vi "Gradient Plot_Raw Image.vi"(8 "error in":errorcluster, 11 "Pixel Column Number":i32=390) -> (0 "error out":errorcluster, 1 "Pixel vs Gradient Graph":cluster{"Y":dbl[], "Y":dbl[]}[](graph), 2 "Pixel vs Intensity Graph":cluster{"Y":dbl[], "Y":dbl[]}[](graph), 3 "Pixel Value":i32, 5 "Maximum Gradient":u8)   [LabVIEW 2016]
uses:
  <vilib>/userdefined/High Color/IMAQdx.ctl
  <vilib>/vision/driver/NI_Vision_Acquisition_Software.lvlib
  <vilib>/vision/NI_Vision_Development_Module.lvlib
panel:
  out "Gradient Array":u8[](array[numeric])
  out "i Array":u8[](array[numeric])
  out "i+1 Array":u8[](array[numeric])
  out "Actual array":u8[](array[numeric])
  out "size(s)":i32
  out "Pixels (U8)":u8[](array[numeric])
  out "Image":T1(plugin-control)
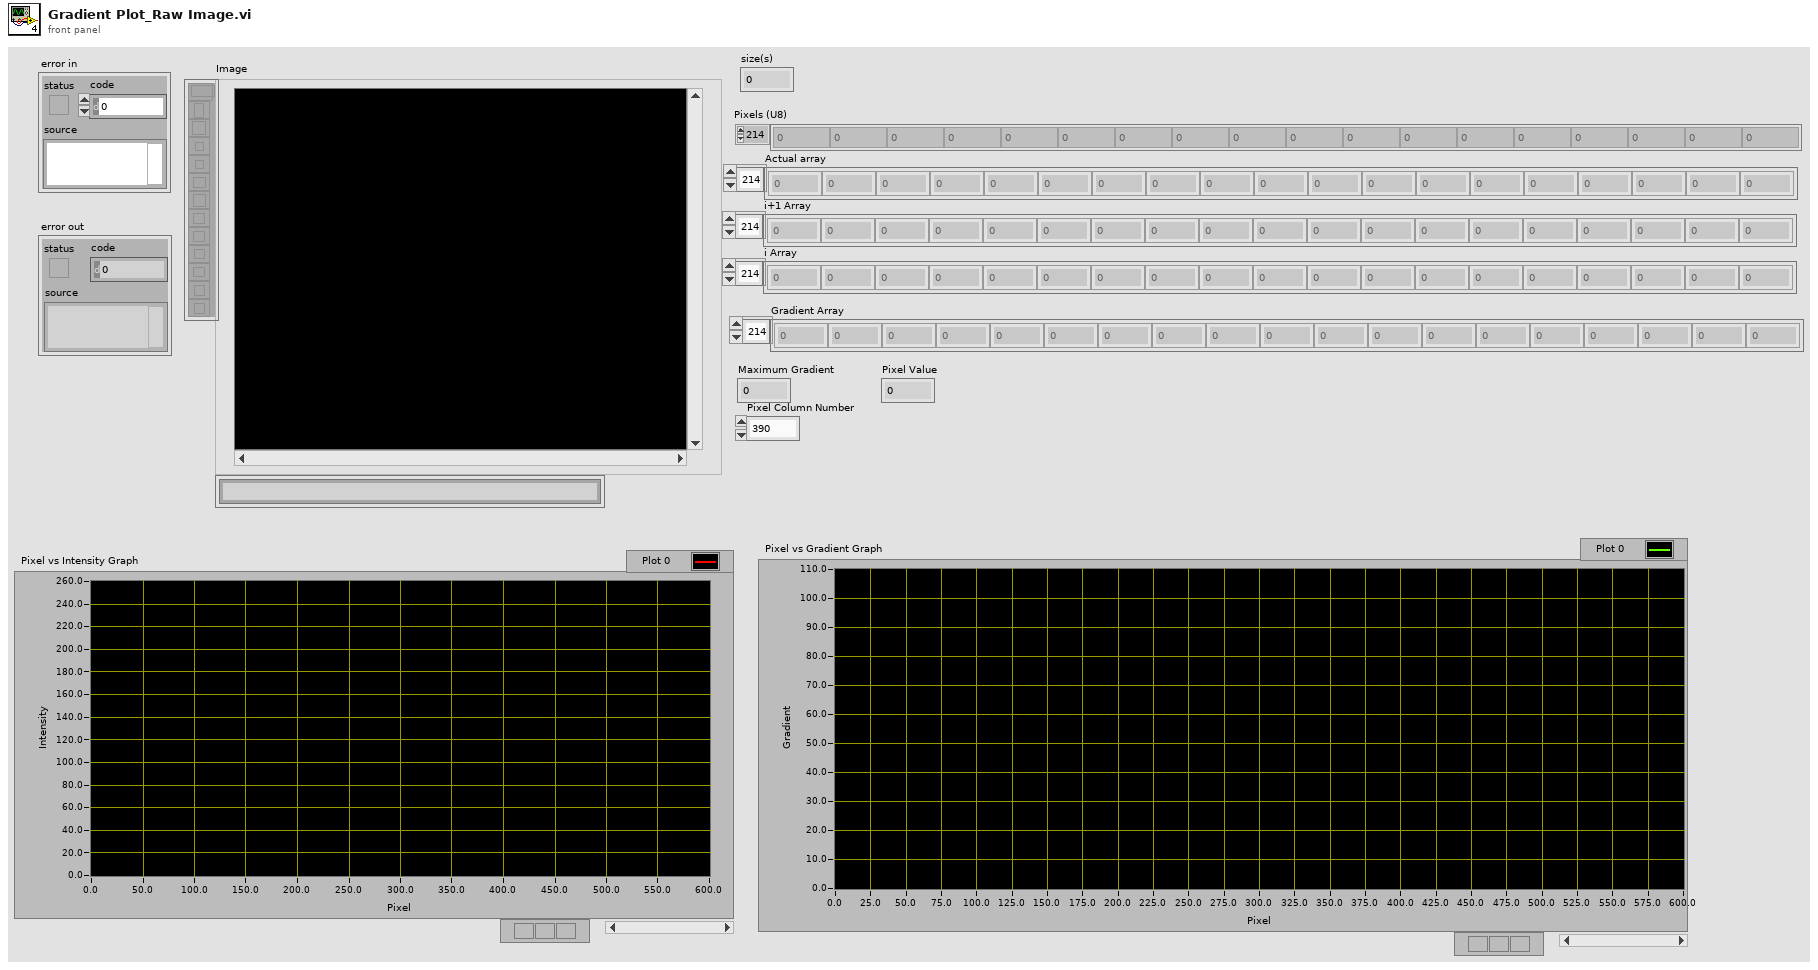
[diagram p1: front panel]
types:
  T1 = typedef "IMAQ Image.ctl" = refnum<image>
  T2 = typedef "IMAQdx.ctl" = refnum<k21>
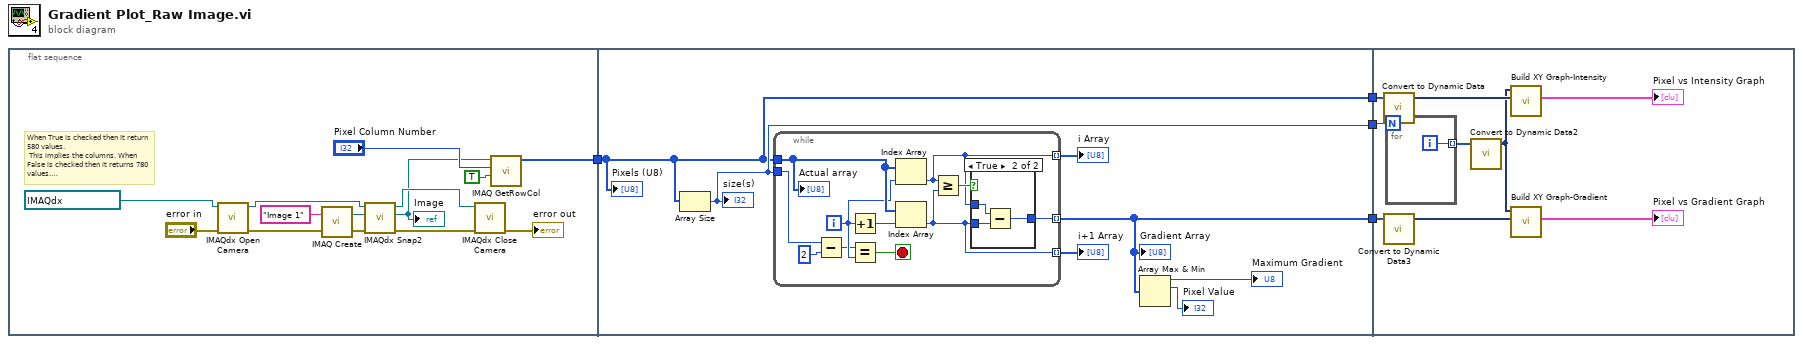
[diagram p0: block diagram]
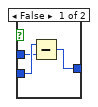
[diagram p2: hidden frame]
diagram:
  n1 = flat-sequence {
    tunnel: [w6] -> w2
    tunnel: [w25] -> w4
    tunnel: [w24] -> w3
    tunnel: w2 -> [w24]
    tunnel: [w21] -> w1
    tunnel: w4 -> [w48]
    tunnel: w3 -> [w49]
    tunnel: w1 -> [w44]
    frame #0 {
      # "When True is checked then it return 580 values.\n This implies the columns. When False is checked then it returns 780 values. \nThis implies rows."
      n2 = call <vilib>:"IMAQdx Open Camera.vi"("error in"="error in", "Session In"=T2 "acA780-75gc") -> ("error out"=w12:errorcluster, "Session Out"=w7:T2)  [unwired: 8 in]
      n3 = call "IMAQ Create"("Image Name"="Image 1", "error in (no error)"=w12) -> ("New Image"=w11:T1, "error out"=w13:errorcluster)  [unwired: 3 in]
      n4 = call <vilib>:"IMAQdx Snap2.vi"("error in"=w13, "Image In"=w11, "Session In"=w7) -> ("error out"=w15:errorcluster, "Image Out"=w5:T1, "Session Out"=w14:T2)  [unwired: 6 in]
      "Image" <- w5
      n5 = call <vilib>:"IMAQdx Close Camera.vi"("error in"=w15, "Session In"=w14) -> ("error out"=→"error out":errorcluster)  [unwired: 9 in]
      n6 = call "IMAQ GetRowCol"("Image"=w5, "Number"="Pixel Column Number", "Row / Column (Row)"=TRUE) -> ("Pixels (U8)"=w6:u8[])  [unwired: 3 in, 4 out]
    }
    frame #1 {
      n7 = Array Size(array=w24) -> (size(s)=w25:i32)
      "size(s)" <- w25
      n8 = while {
        tunnel: w25 -> [w32]
        tunnel: w24 -> [w34]
        tunnel: [w27] -> w23 mode=indexing
        tunnel: [w28] -> w22 mode=indexing
        tunnel: [w26] -> w21 mode=indexing
        i -> [w33]
        stop <- w36 stop-if-true
        n9 = Subtract(x=w32, y=2 ("Number")) -> (x-y=w30:i32)
        n10 = Increment(x=w33) -> (x+1=w35:i32)
        n11 = Equal?(x=w30, y=w33) -> (x = y?=w36:bool)
        n12 = Index Array(array=w34, index=w33) -> (element=w28:u8)
        n13 = Index Array(array=w34, index=w35) -> (element=w27:u8)
        n14 = Greater Or Equal?(x=w28, y=w27) -> (x >= y?=w29:bool)
        n15 = case shown="True" w29 {
          tunnel: w28 -> [w38 w42]
          tunnel: w27 -> [w39 w41]
          tunnel: [w37 w40] -> w26
          frame False {
            n16 = Subtract(x=w39, y=w38) -> (x-y=w37:u8)
          }
          frame True {
            n17 = Subtract(x=w42, y=w41) -> (x-y=w40:u8)
          }
        }
        "Actual array" <- w34
      }
      "i+1 Array" <- w23
      "i Array" <- w22
      "Gradient Array" <- w21
      n18 = Array Max & Min(array=w21) -> (max value=→"Maximum Gradient":u8, max index (indices)=→"Pixel Value":i32)  [unwired: 2 out]
      "Pixels (U8)" <- w24
    }
    frame #2 {
      n19 = call "Convert to Dynamic Data"("Array"=w49) -> ("Dynamic Data Type"=w51:dynamicdata)  [unwired: 3 in]
      n20 = call "Convert to Dynamic Data3"("Array"=w44) -> ("Dynamic Data Type"=w46:dynamicdata)  [unwired: 3 in]
      n21 = for {
        N: w48 -> [_]
        tunnel: [w52] -> w50 mode=indexing
        i -> [w52]
      }
      n22 = call "Convert to Dynamic Data2"("Array"=w50) -> ("Dynamic Data Type"=w47:dynamicdata)  [unwired: 3 in]
      n23 = call "Build XY Graph-Intensity"("Y Input"=w51, "X Input"=w47) -> ("XY Graph"=→"Pixel vs Intensity Graph":cluster{"X":dbl[], "Y":dbl[]}[])  [unwired: 8 in, 1 out]
      n24 = call "Build XY Graph-Gradient"("Y Input"=w46, "X Input"=w47) -> ("XY Graph"=→"Pixel vs Gradient Graph":cluster{"X":dbl[], "Y":dbl[]}[])  [unwired: 8 in, 1 out]
    }
  }
